vi "题目6.vi"() -> ()   [LabVIEW 2017]
panel:
  out "平均数":dbl
  out "波形图":dbl[](graph)
  out "最大值":dbl
  out "最小值":dbl
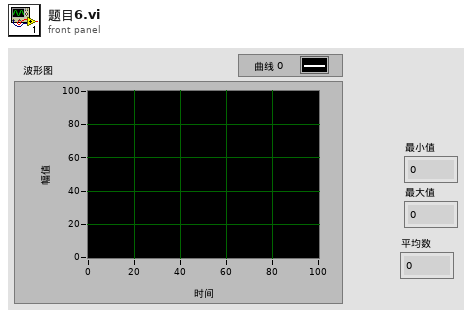
[diagram p1: front panel]
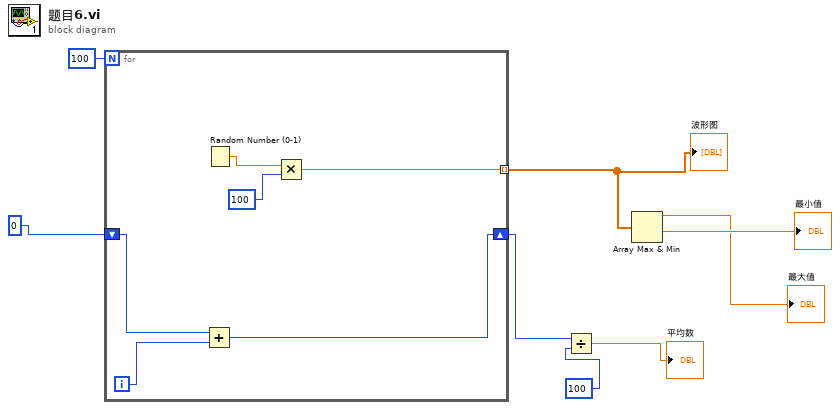
[diagram p0: block diagram]
diagram:
  n1 = for {
    N: 100 -> [_]
    tunnel: [w12] -> w5 mode=indexing
    shift-right: [w9] -> w1
    shift-left: 0 -> [w10]
    i -> [w11]
    n2 = Add(x=w10, y=w11) -> (x+y=w9:i32)
    n3 = Random Number (0-1)() -> (number: 0 to 1=w14:dbl)
    n4 = Multiply(x=w14, y=100) -> (x*y=w12:dbl)
  }
  "波形图" <- w5
  n5 = Divide(x=w1, y=100) -> (x/y=→"平均数":dbl)
  n6 = Array Max & Min(array=w5) -> (max value=→"最大值":dbl, min value=→"最小值":dbl)  [unwired: 2 out]
